vi "limit.vi"(8 "index":dbl, 11 "total":dbl) -> (0 "ind out":dbl)   [LabVIEW 2013]
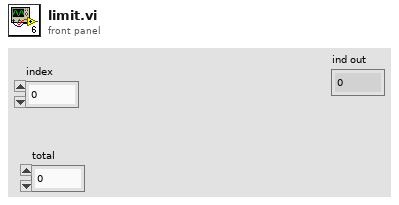
[diagram p1: front panel]
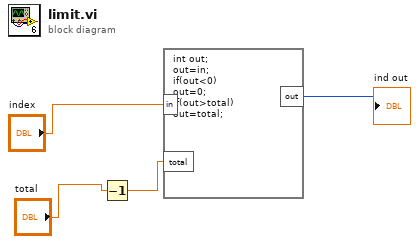
[diagram p0: block diagram]
diagram:
  n1 = Decrement(x="total") -> (x-1=w1:dbl)
  n2 = formula code="int out;\nout=in;\nif(out<0)\nout=0;\nif(out>total)\nout=total;"("in"="index", "total"=w1) -> ("out"=→"ind out":i32)
